vi "LawOfCosines.vi"(1 "Right":dbl, 2 "Opposite":dbl, 3 "Left":dbl) -> (0 "Angle":dbl)   [LabVIEW 2016]
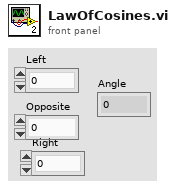
[diagram p1: front panel]
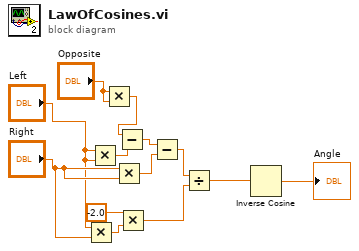
[diagram p0: block diagram]
diagram:
  n1 = Multiply(x="Left", y="Right") -> (x*y=w8:dbl)
  n2 = Multiply(x="Left", y="Left") -> (x*y=w12:dbl)
  n3 = Multiply(x="Opposite", y="Opposite") -> (x*y=w2:dbl)
  n4 = Multiply(x="Right", y="Right") -> (x*y=w11:dbl)
  n5 = Subtract(x=w2, y=w12) -> (x-y=w13:dbl)
  n6 = Multiply(x=-2.0, y=w8) -> (x*y=w9:dbl)
  n7 = Subtract(x=w13, y=w11) -> (x-y=w10:dbl)
  n8 = Divide(x=w10, y=w9) -> (x/y=w4:dbl)
  n9 = Inverse Cosine(1:w4) -> (0:→"Angle":dbl)
